vi "Set pin status.vi"(7 "Value":bool, 8 "error in (no error)":errorcluster, 9 "Pin":dbl, 10 "Port":dbl, 11 "Cypress in":refnum<class "Cypress.lvclass">) -> (0 "error out":errorcluster, 3 "Cypress out":refnum<class "Cypress.lvclass">)   [LabVIEW 2020, in "Cypress.lvclass"]
doc: "Override del papa Set Pin Status"
uses:
  Cypress.lvclass
  5fef197e-7861-4771-90ff-07d51f47743d.vi
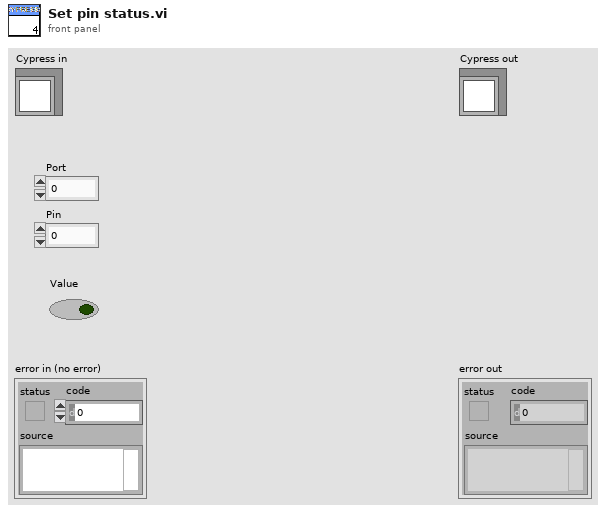
[diagram p1: front panel]
types:
  T1 = typedef "Serial Device.lvclass/serial device brand.ctl" = string
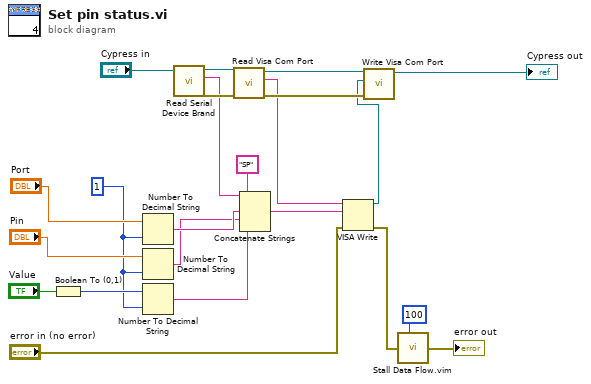
[diagram p0: block diagram]
diagram:
  w1 = i16 1 ("width (-)")
  n1 = Boolean To (0,1)(Boolean="Value") -> (0, 1=w16:i16)
  n2 = Number To Decimal String(number="Port", width (-)=w1) -> (decimal integer string=w11:string)
  n3 = Number To Decimal String(number="Pin", width (-)=w1) -> (decimal integer string=w10:string)
  n4 = Number To Decimal String(number=w16, width (-)=w1) -> (decimal integer string=w9:string)
  n5 = call-dynamic "Read Serial Device Brand.vi"("Serial Device in"="Cypress in") -> ("error out"=w20:errorcluster, "Serial Device Brand"=w12:T1, "Serial Device out"=w23:refnum<class "Cypress.lvclass">)  [unwired: 8 in]
  n6 = call-dynamic "Read Visa Com Port.vi"("error in (no error)"=w20, "Serial Device in"=w23) -> ("error out"=w21:errorcluster, "Visa Com Port"=w13:string, "Serial Device out"=w22:refnum<class "Cypress.lvclass">)  [unwired: 7 in]
  n7 = Concatenate Strings(w12, "SP" ("string"), w11, w10, w9) -> (w14:string)
  n8 = VISA Write(VISA resource name=w13, write buffer=w14, error in (no error)="error in (no error)") -> (VISA resource name out=w4:refnum<visa-resource-name>, error out=w7:errorcluster)  [unwired: 1 out]
  n9 = call-dynamic "Write Visa Com Port.vi"("error in (no error)"=w21, "Visa Com Port"=w4, "Serial Device in"=w22) -> ("Serial Device out"=→"Cypress out":refnum<class "Cypress.lvclass">)  [unwired: 7 in, 1 out]
  n10 = call "Stall Data Flow.vim"("value in"=w7, "milliseconds to wait"=u32 100) -> ("value out"=→"error out":errorcluster)  [unwired: 1 out]
